vi "OFDM-SIM2导频.vi"(1 "输入的OFDM符号":cdb[](array[numeric])) -> (0 "OFDM-IM output":cdb[](array[numeric]))   [LabVIEW 2018]
uses:
  <vilib>/Analysis/1siggen.llb/Ramp Pattern by Samples.vi
  <vilib>/Analysis/NI_AALBase.lvlib
panel:
  out "加导频后":cdb[](array[numeric])
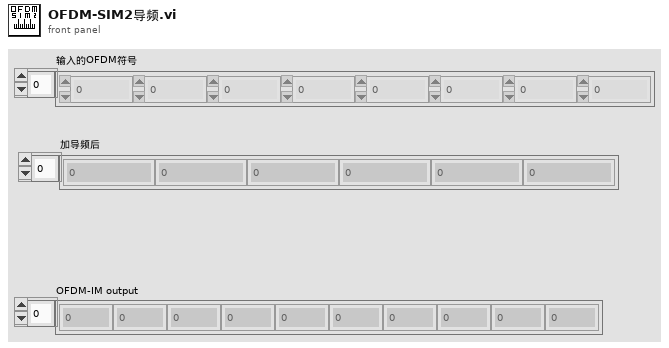
[diagram p1: front panel]
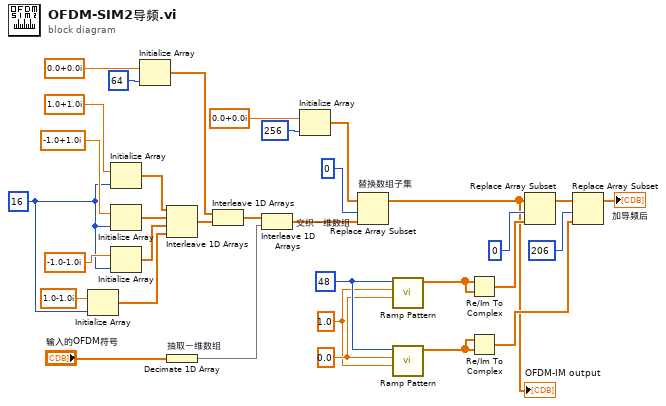
[diagram p0: block diagram]
diagram:
  w2 = 16
  w17 = 1.0
  w18 = 0.0
  w19 = 48
  n1 = Initialize Array(cdb 1.0-1.0i, w2) -> (w8:cdb[])
  n2 = Initialize Array(cdb 1.0+1.0i, w2) -> (w9:cdb[])
  n3 = Initialize Array(cdb -1.0+1.0i, w2) -> (w6:cdb[])
  n4 = Initialize Array(cdb -1.0-1.0i, w2) -> (w7:cdb[])
  n5 = Initialize Array(cdb 0.0+0.0i, 64) -> (w12:cdb[])
  n6 = Interleave 1D Arrays(w9, w6, w7, w8) -> (w1:cdb[])
  n7 = Decimate 1D Array "抽取一维数组"("输入的OFDM符号") -> (w30:cdb[])
  n8 = Interleave 1D Arrays(w12, w1) -> (w11:cdb[])
  n9 = Interleave 1D Arrays "交织一维数组"(w11, w30) -> (w27:cdb[])
  n10 = Initialize Array(cdb 0.0+0.0i ("元素"), 256 ("维数大小")) -> (w29:cdb[])
  n11 = Replace Array Subset "替换数组子集"(array=w29, new element=w27, index=0 ("索引")) -> (w16:cdb[])
  "OFDM-IM output" <- w16
  n12 = call-poly <vilib>:"Ramp Pattern.vi"("start"=w18, "end"=w17, "samples"=w19) -> ("Ramp Pattern"=w26:dbl[])  [unwired: 7 in, 1 out]
  n13 = call-poly <vilib>:"Ramp Pattern.vi"("start"=w17, "end"=w18, "samples"=w19) -> ("Ramp Pattern"=w22:dbl[])  [unwired: 7 in, 1 out]
  n14 = Re/Im To Complex(1:w26, 2:w26) -> (0:w25:cdb[])
  n15 = Re/Im To Complex(1:w22, 2:w22) -> (0:w21:cdb[])
  n16 = Replace Array Subset(array=w16, new element=w25, index=0) -> (w20:cdb[])
  n17 = Replace Array Subset(array=w20, new element=w21, index=206) -> (→"加导频后":cdb[])
